vi "KeyPressLogger.vi"(11 "KeyPressEvent":refnum<user-event>) -> ()   [LabVIEW 2016]
uses:
  <vilib>/Utility/inputDevices.llb/keyboardAcquire.vi
panel:
  out "keys pressed":T1(array[ring])
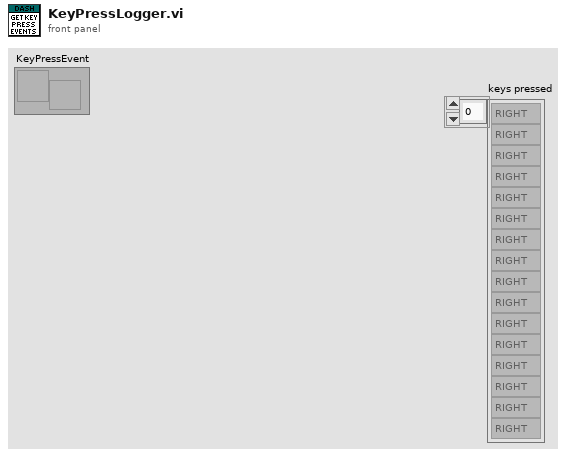
[diagram p1: front panel]
types:
  T1 = enum16{"0", "1", "2", "3", "4", "5", "6", "7", "8", "9", "A", "B", "C", "D", "E", "F", "G", "H", "I", "J", "K", "L", "M", "N", "O", "P", "Q", "R", "S", "T", "U", "V", "W", "X", "Y", "Z", "F1", "F2", "F3", "F4", "F5", "F6", "F7", "F8", "F9", "F10", "F11", "F12", "F13", "F14", "F15", "ADD", "BACK", "BACKSLASH", "CAPITAL", "COMMA", "DECIMAL", "DELETE", "DIVIDE", "DOWN", "END", "EQUALS", "ESCAPE", "GRAVE (`)", "HOME", "INSERT", "LBRACKET", "LCONTROL", "LEFT", "L ALT", "LSHIFT", "LWIN", "MINUS", "MULTIPLY", "NEXT", "NUMLOCK", "NUMPAD_0", "NUMPAD_1", "NUMPAD_2", "NUMPAD_3", "NUMPAD_4", "NUMPAD_5", "NUMPAD_6", "NUMPAD_7", "NUMPAD_8", "NUMPAD_9", "PAUSE", "PERIOD", "PRIOR (PG UP)", "RBRACKET", "RCONTROL", "RETURN", "RIGHT", "R ALT", "RSHIFT", "RWIN", "SCROLL", "SEMICOLON", "SLASH", "SPACE", "SUBTRACT", "TAB", "UP", "ENTER (num pad)", "' (quote)"}[]
  T2 = enum16{"0", "1", "2", "3", "4", "5", "6", "7", "8", "9", "A", "B", "C", "D", "E", "F", "G", "H", "I", "J", "K", "L", "M", "N", "O", "P", "Q", "R", "S", "T", "U", "V", "W", "X", "Y", "Z", "F1", "F2", "F3", "F4", "F5", "F6", "F7", "F8", "F9", "F10", "F11", "F12", "F13", "F14", "F15", "ADD", "BACK", "BACKSLASH", "CAPITAL", "COMMA", "DECIMAL", "DELETE", "DIVIDE", "DOWN", "END", "EQUALS", "ESCAPE", "GRAVE (`)", "HOME", "INSERT", "LBRACKET", "LCONTROL", "LEFT", "L ALT", "LSHIFT", "LWIN", "MINUS", "MULTIPLY", "NEXT", "NUMLOCK", "NUMPAD_0", "NUMPAD_1", "NUMPAD_2", "NUMPAD_3", "NUMPAD_4", "NUMPAD_5", "NUMPAD_6", "NUMPAD_7", "NUMPAD_8", "NUMPAD_9", "PAUSE", "PERIOD", "PRIOR (PG UP)", "RBRACKET", "RCONTROL", "RETURN", "RIGHT", "R ALT", "RSHIFT", "RWIN", "SCROLL", "SEMICOLON", "SLASH", "SPACE", "SUBTRACT", "TAB", "UP", "ENTER (num pad)", "' (quote)"}
  T3 = cluster{bool, bool, bool, cluster{bool, bool, bool, bool, bool}}
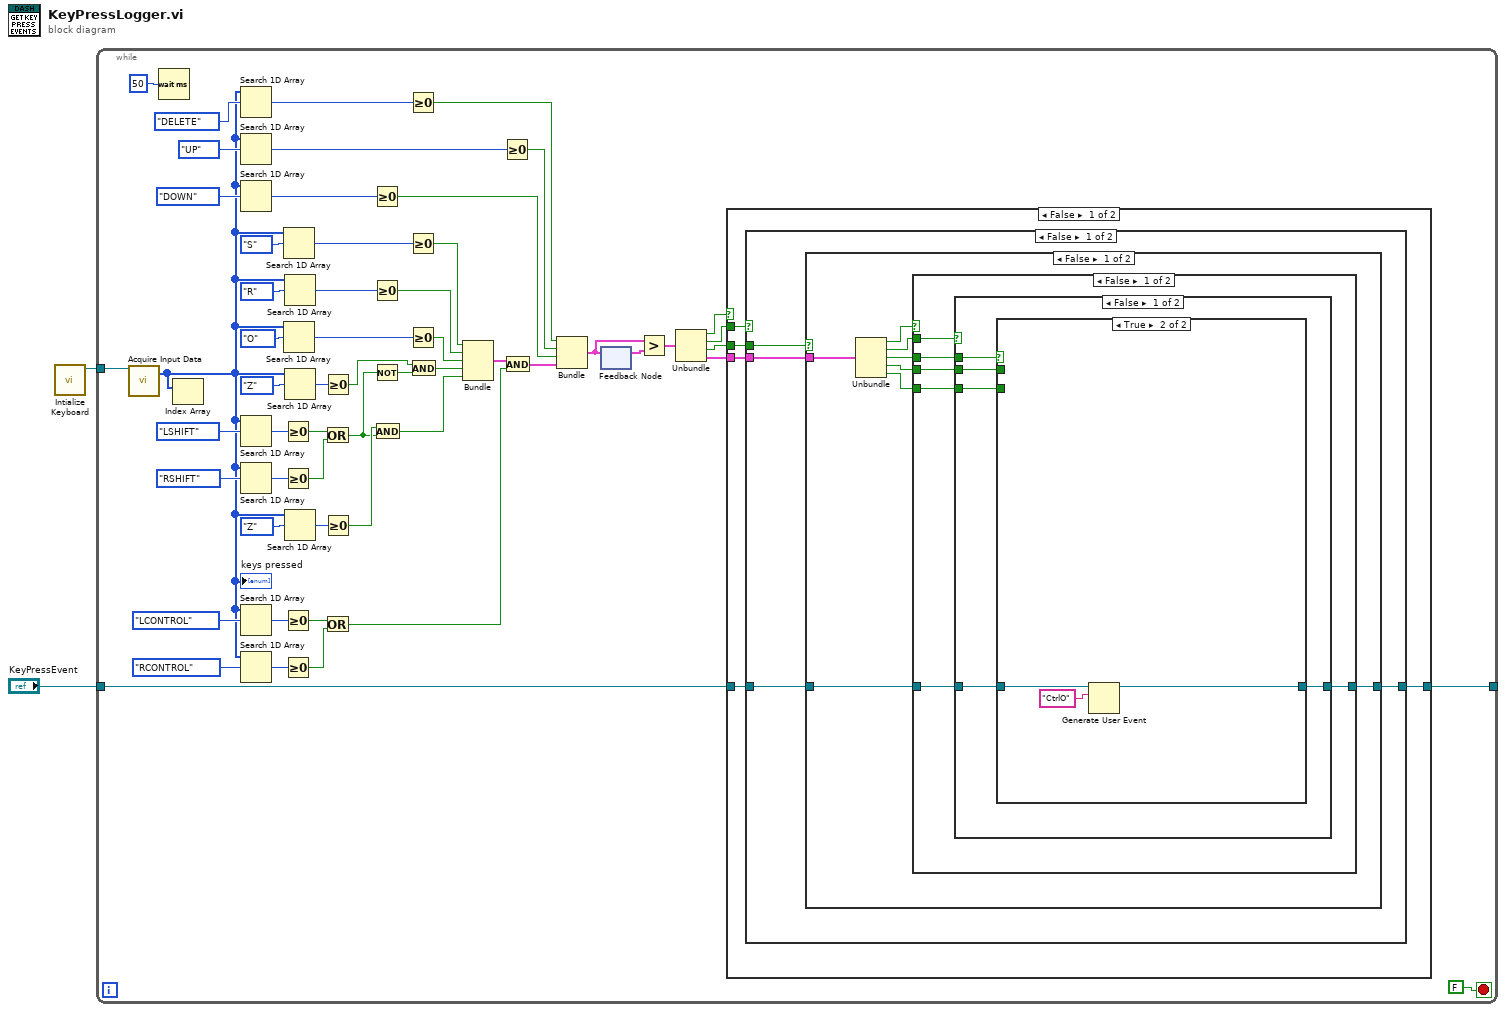
[diagram p0: block diagram]
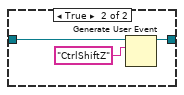
[diagram p3: hidden frame]
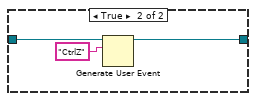
[diagram p4: hidden frame]
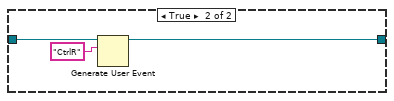
[diagram p5: hidden frame]
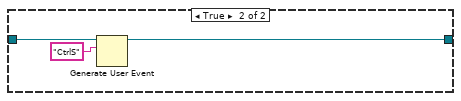
[diagram p6: hidden frame]
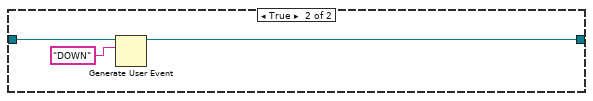
[diagram p7: hidden frame]
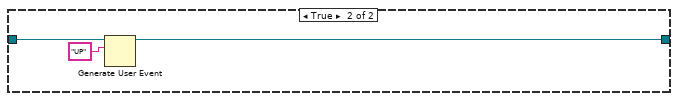
[diagram p8: hidden frame]
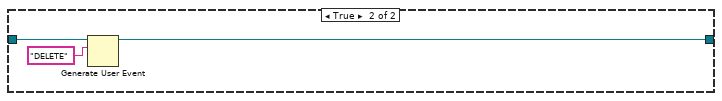
[diagram p9: hidden frame]
diagram:
  n1 = call <vilib>:"Intialize Keyboard.vi"() -> ("device ID"=w2:refnum<k1>)  [unwired: 10 in, 1 out]
  n2 = while {
    tunnel: w2 -> [w57]
    tunnel: "KeyPressEvent" -> [w19]
    tunnel: [w18] -> _
    stop <- FALSE stop-if-true
    n3 = call-poly <vilib>:"Acquire Input Data.vi"("device ID"=w57) -> ("keys pressed"=w20:T1)  [unwired: 16 in, 2 out]
    "keys pressed" <- w20
    n4 = Wait (ms)(milliseconds to wait=u32 50) -> ()  [unwired: 1 out]
    n5 = Index Array(array=w20) -> ()  [unwired: 1 in, 1 out]
    n6 = Search 1D Array(1D array=w20, element=T2."DELETE" ("keyType 3")) -> (index of element=w54:i32)  [unwired: 1 in]
    n7 = Search 1D Array(1D array=w20, element=T2."UP" ("keyType 3")) -> (index of element=w53:i32)  [unwired: 1 in]
    n8 = Search 1D Array(1D array=w20, element=T2."DOWN" ("keyType 3")) -> (index of element=w50:i32)  [unwired: 1 in]
    n9 = Search 1D Array(1D array=w20, element=T2."LSHIFT" ("keyType 3")) -> (index of element=w26:i32)  [unwired: 1 in]
    n10 = Search 1D Array(1D array=w20, element=T2."RSHIFT" ("keyType 3")) -> (index of element=w27:i32)  [unwired: 1 in]
    n11 = Search 1D Array(1D array=w20, element=T2."LCONTROL" ("keyType 3")) -> (index of element=w48:i32)  [unwired: 1 in]
    n12 = Search 1D Array(1D array=w20, element=T2."RCONTROL" ("keyType 3")) -> (index of element=w47:i32)  [unwired: 1 in]
    n13 = Greater Or Equal To 0?(x=w26) -> (x >= 0?=w29:bool)
    n14 = Greater Or Equal To 0?(x=w27) -> (x >= 0?=w30:bool)
    n15 = Greater Or Equal To 0?(x=w48) -> (x >= 0?=w45:bool)
    n16 = Greater Or Equal To 0?(x=w47) -> (x >= 0?=w44:bool)
    n17 = Search 1D Array(1D array=w20, element=T2."S" ("keyType 3")) -> (index of element=w43:i32)  [unwired: 1 in]
    n18 = Search 1D Array(1D array=w20, element=T2."O" ("keyType 3")) -> (index of element=w39:i32)  [unwired: 1 in]
    n19 = Search 1D Array(1D array=w20, element=T2."R" ("keyType 3")) -> (index of element=w40:i32)  [unwired: 1 in]
    n20 = Search 1D Array(1D array=w20, element=T2."Z" ("keyType 3")) -> (index of element=w21:i32)  [unwired: 1 in]
    n21 = Search 1D Array(1D array=w20, element=T2."Z" ("keyType 3")) -> (index of element=w31:i32)  [unwired: 1 in]
    n22 = Greater Or Equal To 0?(x=w21) -> (x >= 0?=w17:bool)
    n23 = Or(x=w29, y=w30) -> (x .or. y?=w14:bool)
    n24 = Greater Or Equal To 0?(x=w31) -> (x >= 0?=w24:bool)
    n25 = Or(x=w45, y=w44) -> (x .or. y?=w34:bool)
    n26 = Greater Or Equal To 0?(x=w50) -> (x >= 0?=w12:bool)
    n27 = Greater Or Equal To 0?(x=w40) -> (x >= 0?=w36:bool)
    n28 = Not(x=w14) -> (.not. x?=w15:bool)
    n29 = And(x=w24, y=w14) -> (x .and. y?=w23:bool)
    n30 = Greater Or Equal To 0?(x=w54) -> (x >= 0?=w10:bool)
    n31 = Greater Or Equal To 0?(x=w43) -> (x >= 0?=w35:bool)
    n32 = Greater Or Equal To 0?(x=w39) -> (x >= 0?=w37:bool)
    n33 = And(x=w17, y=w15) -> (x .and. y?=w16:bool)
    n34 = Bundle(w35, w36, w37, w16, w23) -> (w33:cluster{bool, bool, bool, bool, bool})  [unwired: 1 in]
    n35 = Greater Or Equal To 0?(x=w53) -> (x >= 0?=w11:bool)
    n36 = And(x=w33, y=w34) -> (x .and. y?=w13:cluster{bool, bool, bool, bool, bool})
    n37 = Bundle(w10, w11, w12, w13) -> (w9:T3)  [unwired: 1 in]
    n38 = feedback-in #1(w9) -> ()
    n39 = feedback #1() -> (w8:T3)  [unwired: 1 in]
    n40 = Greater?(x=w9, y=w8) -> (0:w7:T3)
    n41 = Unbundle(w7) -> (w6:bool, w5:bool, w4:bool, w3:cluster{bool, bool, bool, bool, bool})
    n42 = case shown="False" w6 {
      tunnel: w5 -> [w63 _]
      tunnel: w4 -> [w62 _]
      tunnel: w3 -> [w61 _]
      tunnel: w19 -> [w60 w117]
      tunnel: [w59 w116] -> w18
      frame False {
        n43 = case shown="False" w63 {
          tunnel: w62 -> [w67 _]
          tunnel: w61 -> [w66 _]
          tunnel: w60 -> [w65 w114]
          tunnel: [w64 w113] -> w59
          frame False {
            n44 = case shown="False" w67 {
              tunnel: w66 -> [w75 _]
              tunnel: w65 -> [w69 w111]
              tunnel: [w68 w110] -> w64
              frame False {
                n45 = Unbundle(w75) -> (w74:bool, w73:bool, w72:bool, w71:bool, w70:bool)
                n46 = case shown="False" w74 {
                  tunnel: w73 -> [w81 _]
                  tunnel: w72 -> [w80 _]
                  tunnel: w71 -> [w79 _]
                  tunnel: w70 -> [w78 _]
                  tunnel: w69 -> [w77 w108]
                  tunnel: [w76 w107] -> w68
                  frame False {
                    n47 = case shown="False" w81 {
                      tunnel: w80 -> [w86 _]
                      tunnel: w79 -> [w85 _]
                      tunnel: w78 -> [w84 _]
                      tunnel: w77 -> [w83 w105]
                      tunnel: [w82 w104] -> w76
                      frame False {
                        n48 = case shown="True" w86 {
                          tunnel: w85 -> [w90 _]
                          tunnel: w84 -> [w89 _]
                          tunnel: w83 -> [w88 w102]
                          tunnel: [w87 w101] -> w82
                          frame False {
                            n49 = case shown="False" w90 {
                              tunnel: w89 -> [w93 _]
                              tunnel: w88 -> [w92 w100]
                              tunnel: [w91 w98] -> w87
                              frame False {
                                n50 = case shown="False" w93 {
                                tunnel: w92 -> [w94 w97]
                                tunnel: [w94 w95] -> w91
                                frame False {
                                }
                                frame True {
                                n51 = Generate User Event(user event=w97, event data cluster="CtrlShiftZ" ("event data")) -> (user event out=w95:refnum<user-event>)  [unwired: 2 in, 1 out]
                                }
                                }
                              }
                              frame True {
                                n52 = Generate User Event(user event=w100, event data cluster="CtrlZ" ("event data")) -> (user event out=w98:refnum<user-event>)  [unwired: 2 in, 1 out]
                              }
                            }
                          }
                          frame True {
                            n53 = Generate User Event(user event=w102, event data cluster="CtrlO" ("event data")) -> (user event out=w101:refnum<user-event>)  [unwired: 2 in, 1 out]
                          }
                        }
                      }
                      frame True {
                        n54 = Generate User Event(user event=w105, event data cluster="CtrlR" ("event data")) -> (user event out=w104:refnum<user-event>)  [unwired: 2 in, 1 out]
                      }
                    }
                  }
                  frame True {
                    n55 = Generate User Event(user event=w108, event data cluster="CtrlS" ("event data")) -> (user event out=w107:refnum<user-event>)  [unwired: 2 in, 1 out]
                  }
                }
              }
              frame True {
                n56 = Generate User Event(user event=w111, event data cluster="DOWN" ("event data")) -> (user event out=w110:refnum<user-event>)  [unwired: 2 in, 1 out]
              }
            }
          }
          frame True {
            n57 = Generate User Event(user event=w114, event data cluster="UP" ("event data")) -> (user event out=w113:refnum<user-event>)  [unwired: 2 in, 1 out]
          }
        }
      }
      frame True {
        n58 = Generate User Event(user event=w117, event data cluster="DELETE" ("event data")) -> (user event out=w116:refnum<user-event>)  [unwired: 2 in, 1 out]
      }
    }
  }
